vi "CABLE_SetCuff_Thigh.vi"(9 "Extra Weight (kg)":dbl, 10 "Upper Cuff to Lower Cuff (m)":dbl, 11 "Lower Cuff to Knee (m)":dbl) -> (2 "Thigh Cuff Low":T1={"BodyID"=0, "CoM(CuffCS)"={"Coord4"=[0.0, 0.0, 0.0, 1.0], "ID"=0}, "Mass(kg)"=0.0, "CablePts(CuffCS)"=[], "Cuff->Body"=[[1.0, 0.0, 0.0, 0.0], [0.0, 1.0, 0.0, 0.0], [0.0, 0.0, 1.0, 0.0], [0.0, 0.0, 0.0, 1.0]]}, 3 "Thigh Cuff High":T1={"BodyID"=0, "CoM(CuffCS)"={"Coord4"=[0.0, 0.0, 0.0, 1.0], "ID"=0}, "Mass(kg)"=0.0, "CablePts(CuffCS)"=[], "Cuff->Body"=[[1.0, 0.0, 0.0, 0.0], [0.0, 1.0, 0.0, 0.0], [0.0, 0.0, 1.0, 0.0], [0.0, 0.0, 0.0, 1.0]]})   [LabVIEW 2016, in "CAlex2.lvclass"]
uses:
  CAlex2.lvclass
  SerialChain-Cable/TypeDef/Cuff.ctl
  SerialChain/TypeDef/PointOnBody.ctl
  <vilib>/Analysis/Matrix/Datatypes/RealMatrix.ctl
  SerialChain/TypeDef/xyzO.ctl
  <vilib>/Analysis/Matrix/NI_Matrix.lvlib
  SerialChain/SerialChain.lvclass
  SerialChain-Cable/SerialChain-Cable.lvclass
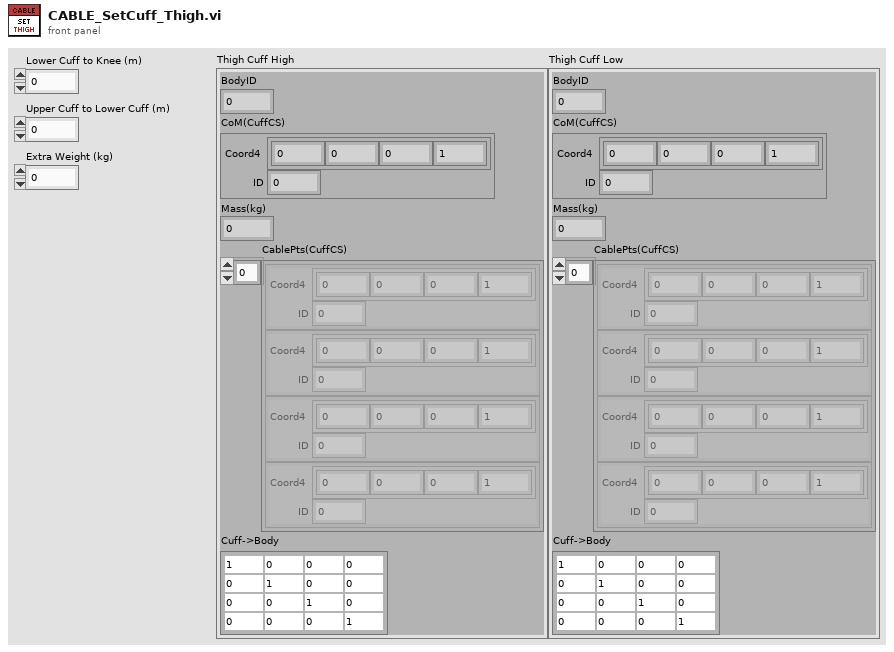
[diagram p1: front panel]
types:
  T1 = typedef "SerialChain-Cable.lvclass/Cuff.ctl" = cluster{"BodyID":i32, "CoM(CuffCS)":T2, "Mass(kg)":dbl, "CablePts(CuffCS)":T2[], "Cuff->Body":T3}
  T2 = typedef "SerialChain.lvclass/PointOnBody.ctl" = cluster{"Coord4":dbl[], "ID":i32}
  T3 = typedef "NI_Matrix.lvlib/RealMatrix.ctl" = dbl[][]
  T4 = typedef "SerialChain.lvclass/xyzO.ctl" = enum16{"X", "Y", "Z", "O"}
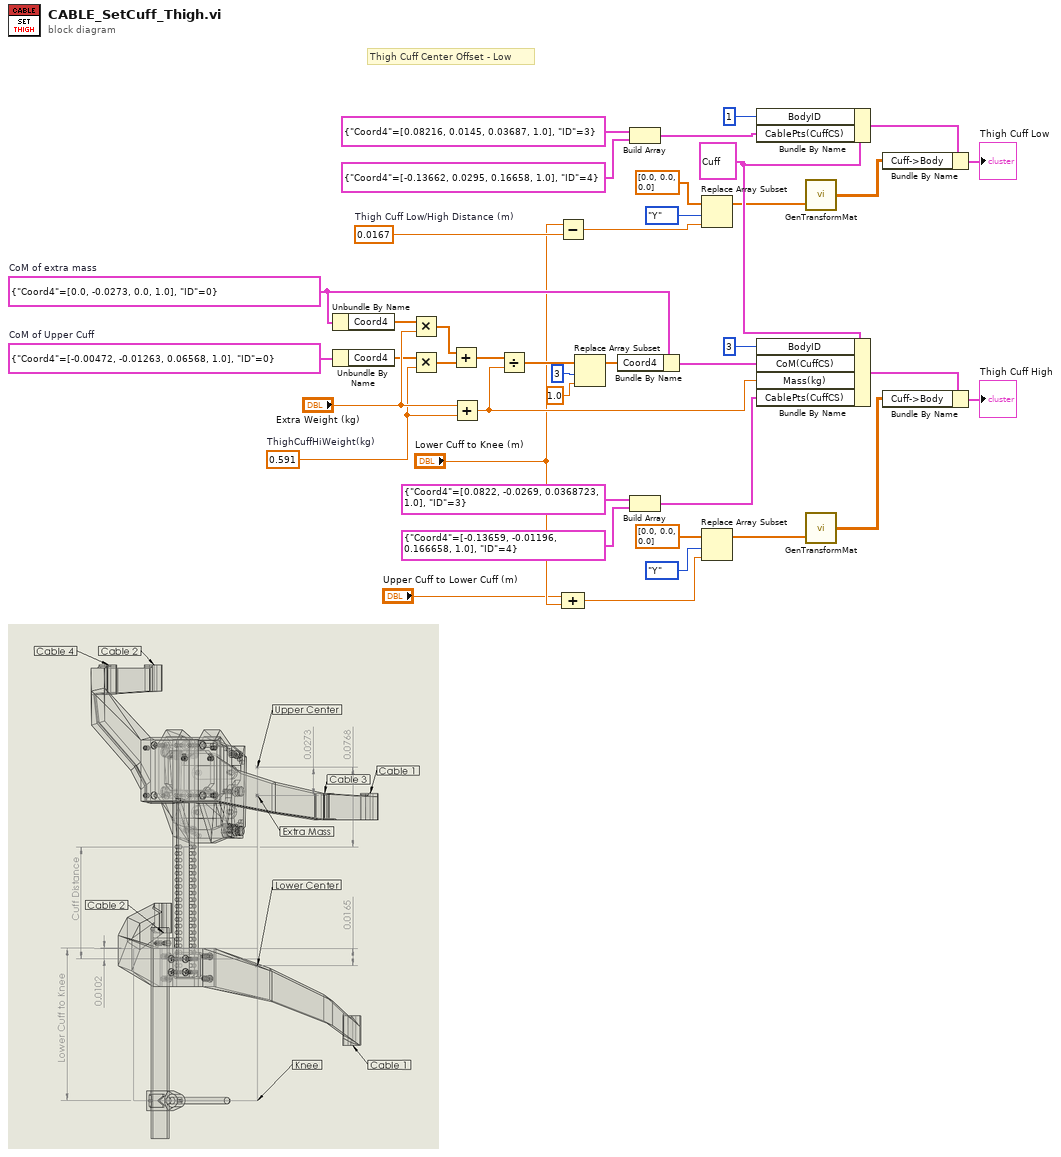
[diagram p0: block diagram]
diagram:
  w15 = 0.0167  # Thigh Cuff Low/High Distance (m)
  w24 = T2 {"Coord4"=[0.0, -0.0273, 0.0, 1.0], "ID"=0}  # CoM of extra mass
  w29 = 0.591  # ThighCuffHiWeight(kg)
  w33 = T2 {"Coord4"=[-0.00472, -0.01263, 0.06568, 1.0], "ID"=0}  # CoM of Upper Cuff
  w18 = T1 {"BodyID"=0, "CoM(CuffCS)"={"Coord4"=[0.0, 0.0, 0.0, 1.0], "ID"=0}, "Mass(kg)"=0.0, "CablePts(CuffCS)"=[], "Cuff->Body"=[[1.0, 0.0, 0.0, 0.0], [0.0, 1.0, 0.0, 0.0], [0.0, 0.0, 1.0, 0.0], [0.0, 0.0, 0.0, 1.0]]} ("Cuff Design")
  # "Thigh Cuff Center Offset - Low"
  n1 = Unbundle By Name(w24) -> ("Coord4"=w32:dbl[])
  n2 = Unbundle By Name(w33) -> ("Coord4"=w30:dbl[])
  n3 = Multiply(x=w32, y="Extra Weight (kg)") -> (x*y=w28:dbl[])
  n4 = Multiply(x=w30, y=w29) -> (x*y=w27:dbl[])
  n5 = Add(x=w28, y=w27) -> (x+y=w26:dbl[])
  n6 = Add(x="Extra Weight (kg)", y=w29) -> (x+y=w25:dbl)
  n7 = Divide(x=w26, y=w25) -> (x/y=w22:dbl[])
  n8 = Subtract(x="Lower Cuff to Knee (m)", y=w15) -> (x-y=w9:dbl)
  n9 = Compound Arithmetic op=ADD("Upper Cuff to Lower Cuff (m)", "Lower Cuff to Knee (m)") -> (w5:dbl)
  n10 = Replace Array Subset(array=w22, new element=1.0 ("new element/subarray"), index=3) -> (w21:dbl[])
  n11 = Bundle By Name(cluster=w24, "Coord4"=w21) -> (w23:T2)
  n12 = Build Array(T2 {"Coord4"=[0.08216, 0.0145, 0.03687, 1.0], "ID"=3} ("CoM(CuffCS)"), T2 {"Coord4"=[-0.13662, 0.0295, 0.16658, 1.0], "ID"=4} ("CoM(CuffCS)")) -> (w35:T2[])
  n13 = Build Array(T2 {"Coord4"=[0.0822, -0.0269, 0.0368723, 1.0], "ID"=3} ("CoM(CuffCS)"), T2 {"Coord4"=[-0.13659, -0.01196, 0.166658, 1.0], "ID"=4} ("CoM(CuffCS)")) -> (w38:T2[])
  n14 = Replace Array Subset(array=dbl[] [0.0, 0.0, 0.0], new element=w9, index=xyzO."Y" ("XYZ")) -> (w11:dbl[])
  n15 = Replace Array Subset(array=dbl[] [0.0, 0.0, 0.0], new element=w5, index=xyzO."Y" ("XYZ")) -> (w4:dbl[])
  n16 = Bundle By Name(cluster=w18, "BodyID"=1, "CablePts(CuffCS)"=w35) -> (w17:T1)
  n17 = Bundle By Name(cluster=w18, "BodyID"=3, "CoM(CuffCS)"=w23, "Mass(kg)"=w25, "CablePts(CuffCS)"=w38) -> (w16:T1)
  n18 = call "GenTransformMat.vi"("Translate 3Vector"=w11) -> ("Transformation Matrix"=w13:T3)  [unwired: 1 in]
  n19 = call "GenTransformMat.vi"("Translate 3Vector"=w4) -> ("Transformation Matrix"=w3:T3)  [unwired: 1 in]
  n20 = Bundle By Name(cluster=w17, "Cuff->Body"=w13) -> (→"Thigh Cuff Low":T1)
  n21 = Bundle By Name(cluster=w16, "Cuff->Body"=w3) -> (→"Thigh Cuff High":T1)
